vi "Control Panel.vi"(8 "error in (no error)":errorcluster, 11 "Spectrometer Triax 550 in":refnum<class "Spectrometer Triax 550.lvclass">) -> (0 "error out":errorcluster, 3 "Spectrometer Triax 550 out":refnum<class "Spectrometer Triax 550.lvclass">)   [LabVIEW 2023, in "Spectrometer Triax 550.lvclass"]
uses:
  Spectrometer Triax 550.lvclass
  JY-SPEX-TRIAX/controls.llb/Turret Position (TRIAX).ctl
  <vilib>/Utility/error.llb/DialogType.ctl
  JY-SPEX-TRIAX/controls.llb/Slits.ctl
  Spectrometer Triax 550.lvclass/Spectrometer Triax 550.ctl
  JY-SPEX-TRIAX/JY-SPEX-TRIAX.lvlib
  Utility Classes/Scannable/Scannable.lvclass
panel:
  out "?":bool
  out "Title 2":string="Spectrometer Control Program"
  in  "Select Grating":T1
  out "Construct":bool
  out "Init":T2
  out "Status":string
  in  "Shutter":bool
  in  "Set Mirror":bool
  in  "Exit Mirror Pos":bool=TRUE
  in  "Exit":bool
  out "Ready (when flashing)":bool
  out "Slits Open?":bool
  in  "Close Slits":bool
  in  "stepsize":dbl[unit]
  in  "Optimize":bool
  out "groovedensity":dbl[unit] caption="Groove Density"
  out "blazewave":dbl[unit] caption="Blaze Wavelength"
  in  "Set Turret":bool
  out "Title":string="Spectrometer Control Program"
  in  "Reset":bool
  out "Current Wavelength":dbl[unit]
  in  "Target Wavelength":dbl[unit]=4.0000000000000003e-07 min=0.0 max=1.4000000000000001e-06 step=1.0000000000000002e-10
  in  "Jump To Wavelength":bool
  in  "Set Slits":bool
  out "currentlat":dbl[unit] format="%#_6f"
  out "currentaxial":dbl[unit] format="%#_6f"
  in  "gotolat":dbl[unit] min=0.0 max=0.0022 step=1e-05
  in  "gotoaxial":dbl[unit] min=0.0 max=0.0022 step=1e-05 format="%#_6f"
  # "Grating A"
  # "Initialization"
  # "Wavelength Control"
  # "Turret and Other Specs\n(initial mirror value may be incorrect!)"
  # "Grating B"
  # "Slit Widths"
  # "Target"
  # "Current"
  # "AXIAL/CCD"
  # "LATERAL/PMT"
  # "Axial Entrance"
  # "Lateral Exit"
  # "(will round to nearest step size - 2 µm)"
  # "Grating C"
  # "NOTE: initial shutter value may be incorrect!  Toggle switch to set a definite value."
  # "Grooves/mm       Blaze           Cal Offset\nGrating A           1200           500 nm            -35571\nGrating B           1200           750 nm            -38317\nGrating C             600         1000 nm           -40000 (??)"
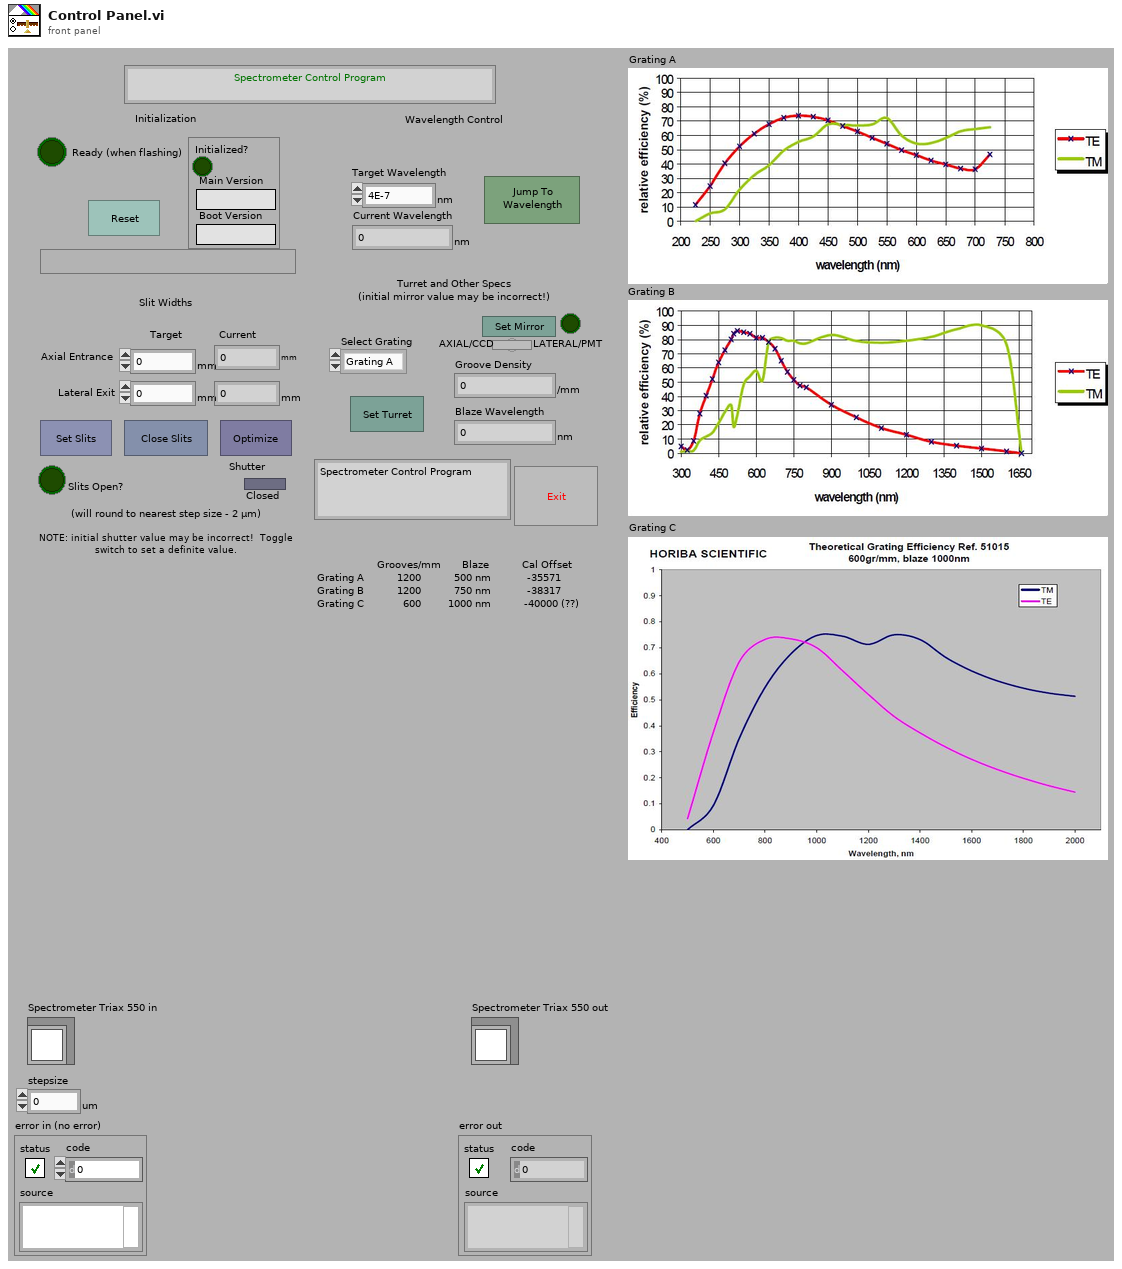
[diagram p1: front panel]
types:
  T1 = typedef "JY-SPEX-TRIAX.lvlib/Turret Position (TRIAX).ctl" = enum16{"Grating A", "Grating B", "Grating C"}
  T2 = cluster{"Initialized?":bool, "Main Version":string, "Boot Version":string, "Spectrometer Number":enum16{"Zero", "One"}}
  T3 = typedef "JY-SPEX-TRIAX.lvlib/Slits.ctl" = enum16{"0 (Front/Axial Entrance)", "1 (Side/Lateral Entrance)", "2 (Front/Axial Exit)", "3 (Side/Lateral Exit)"}
  T4 = typedef "DialogType.ctl" = u16
  T5 = typedef "JY-SPEX-TRIAX.lvlib/Monochromator System Number.ctl" = enum16{"Zero", "One"}
  T6 = cluster{"Initialized?":bool, "Main Version":string, "Boot Version":string, "Mono System #":T5}
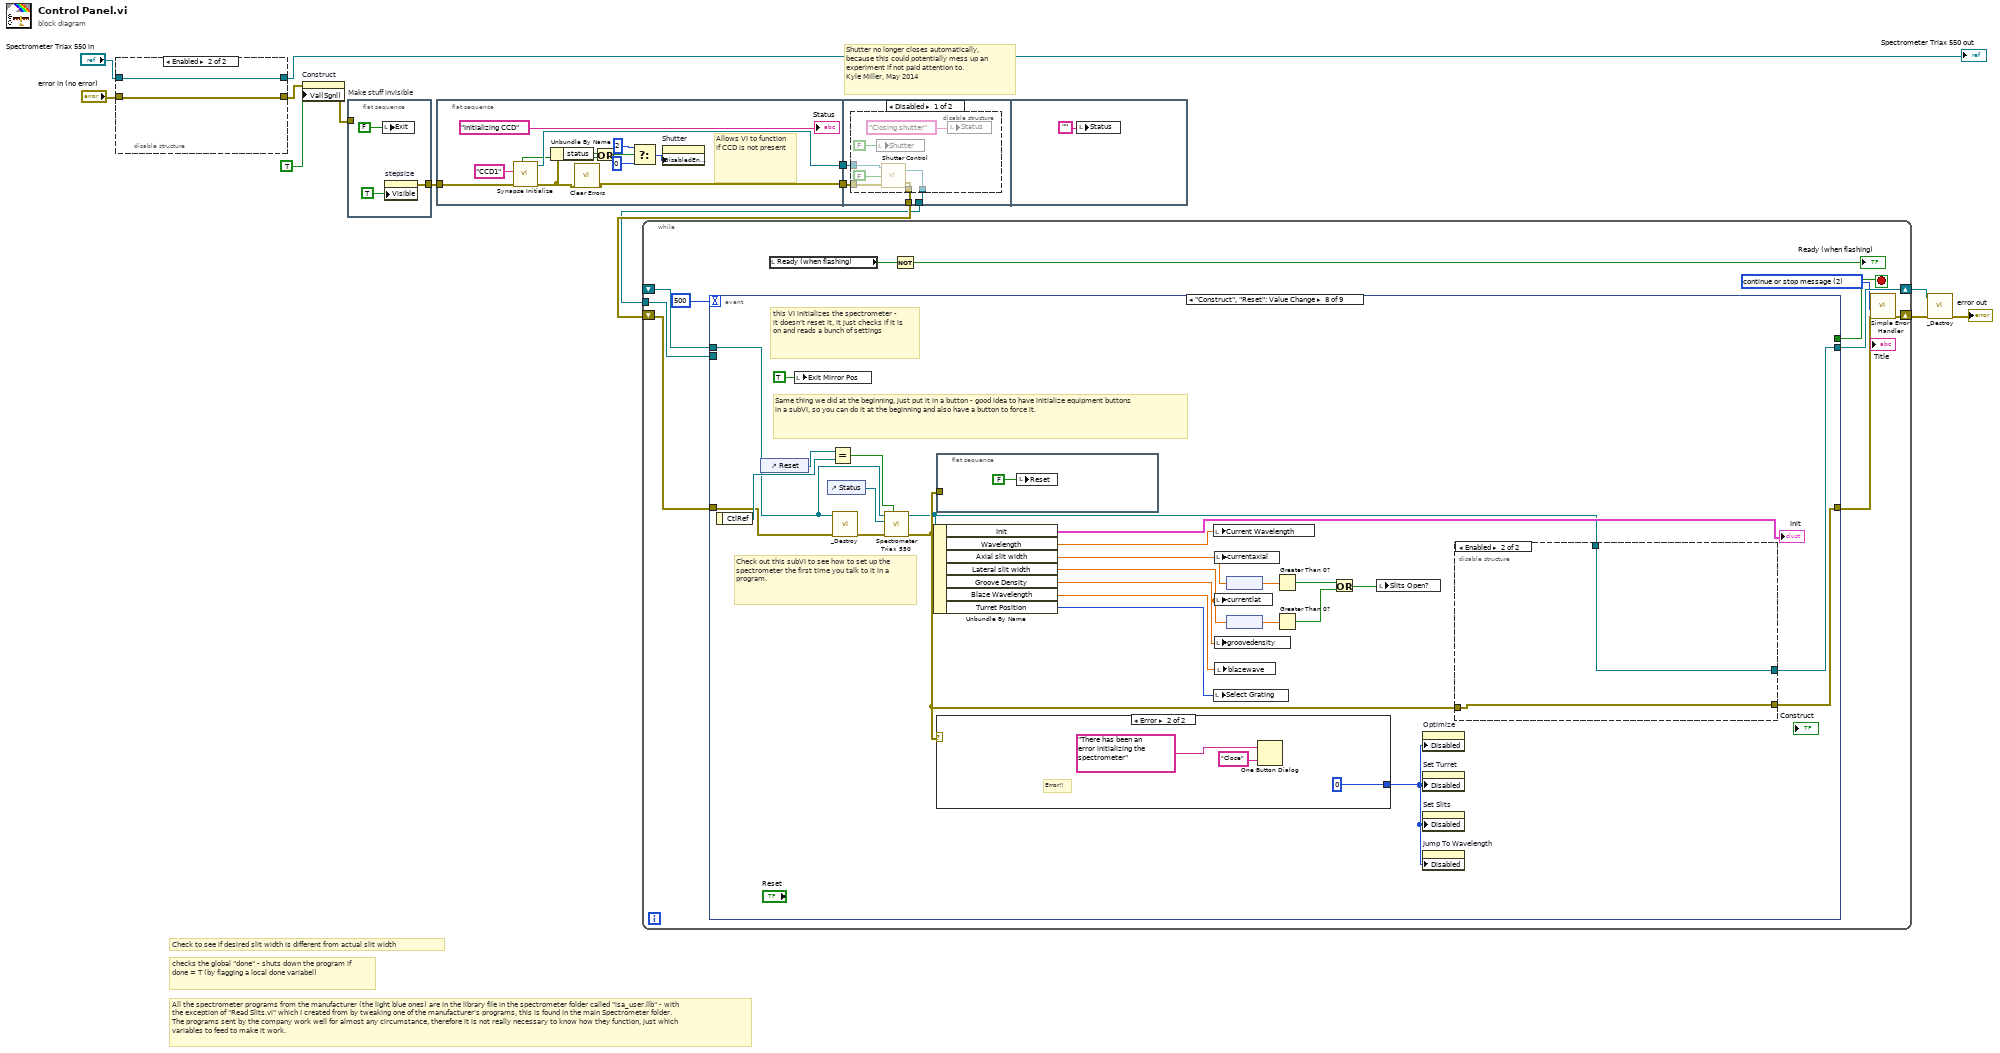
[diagram p0: block diagram]
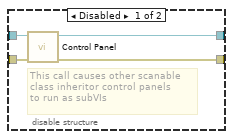
[diagram p2: hidden frame]
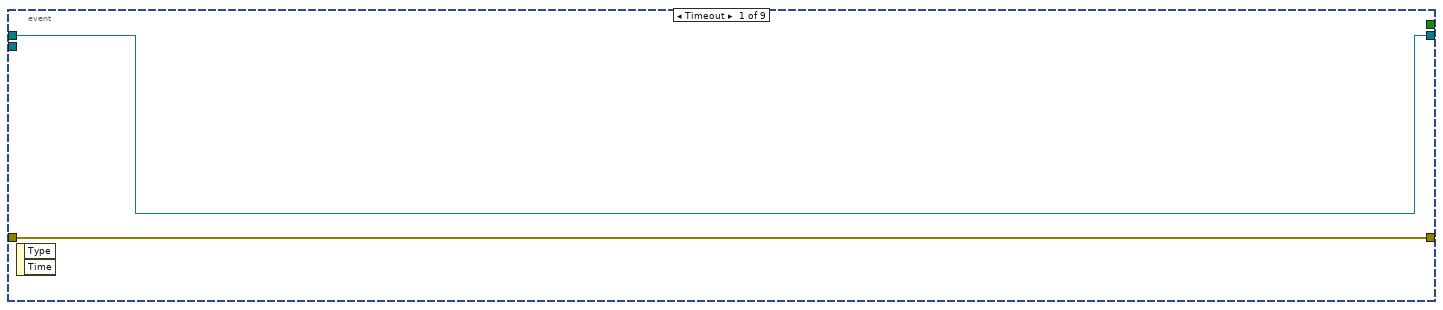
[diagram p4: hidden frame]
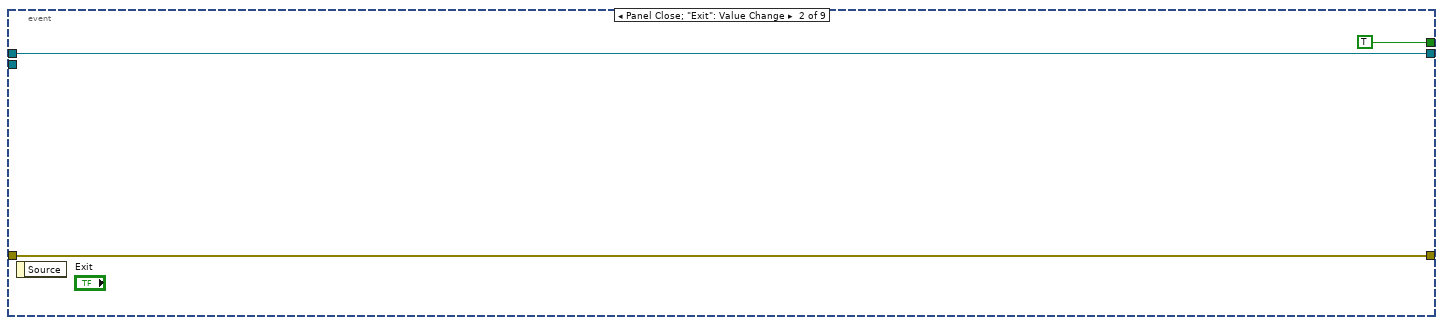
[diagram p5: hidden frame]
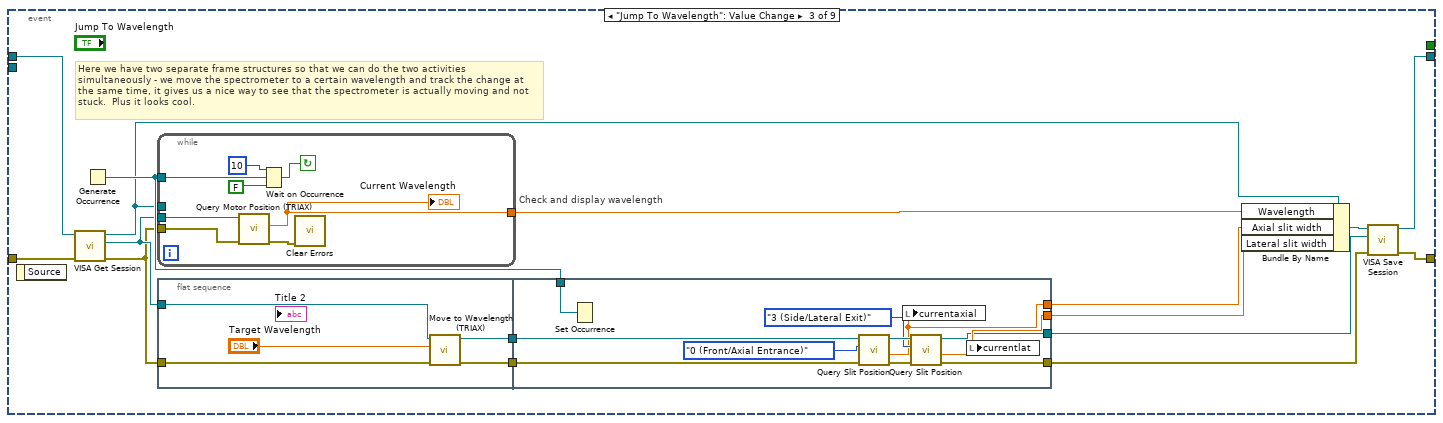
[diagram p6: hidden frame]
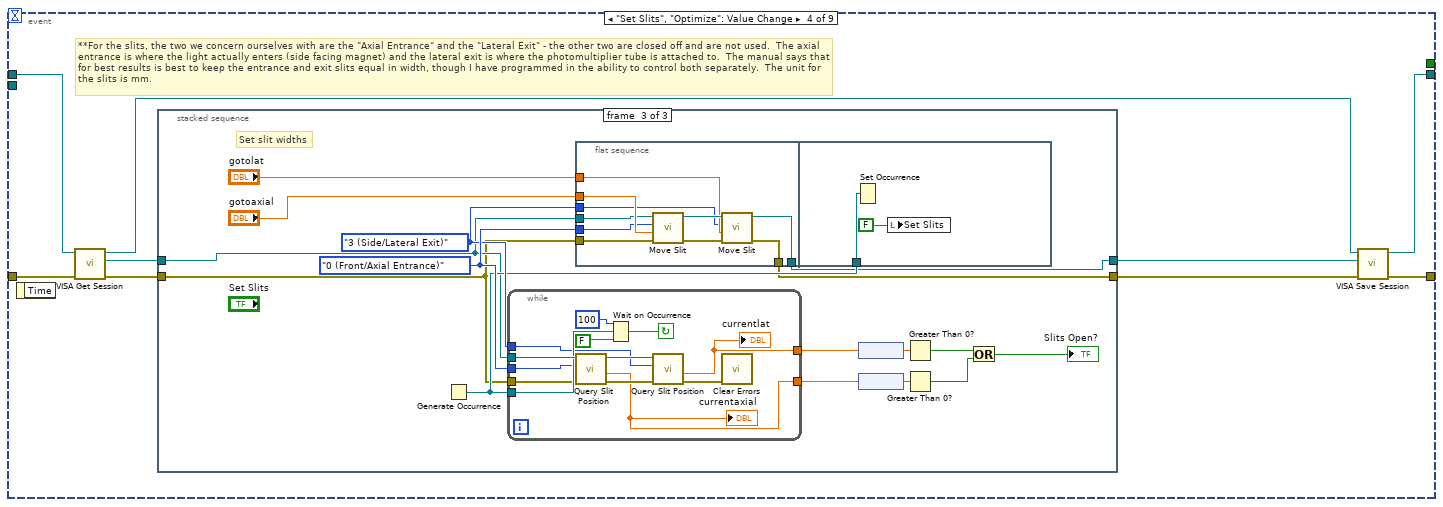
[diagram p7: hidden frame]
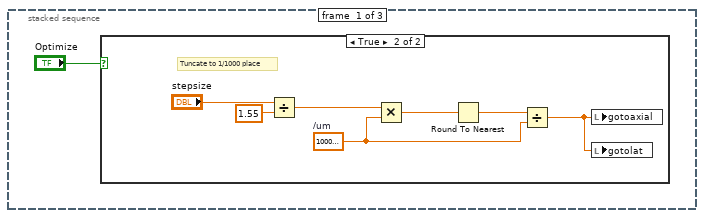
[diagram p8: hidden frame]
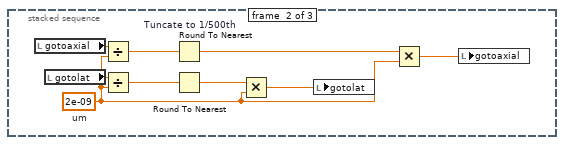
[diagram p10: hidden frame]
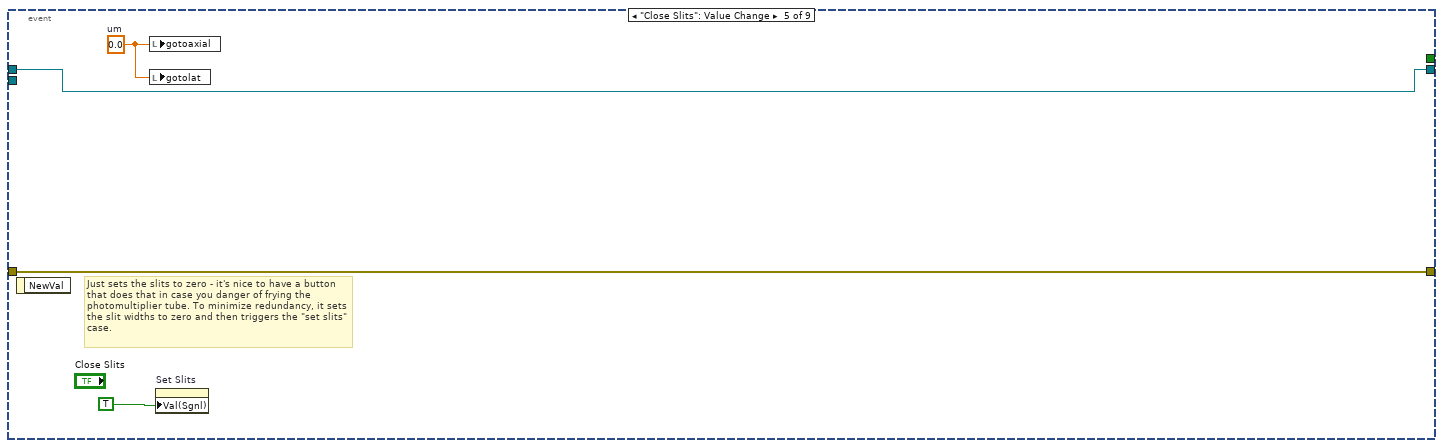
[diagram p11: hidden frame]
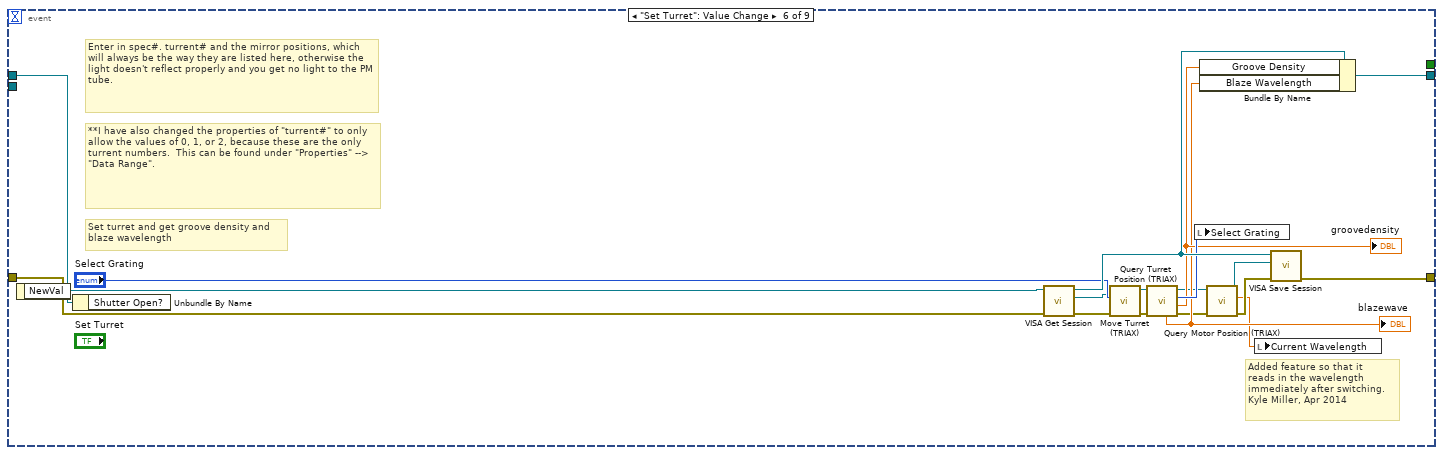
[diagram p12: hidden frame]
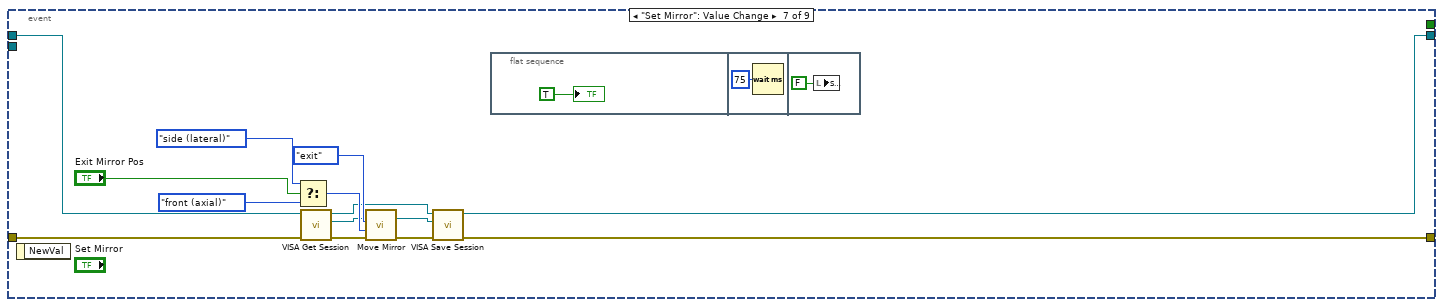
[diagram p13: hidden frame]
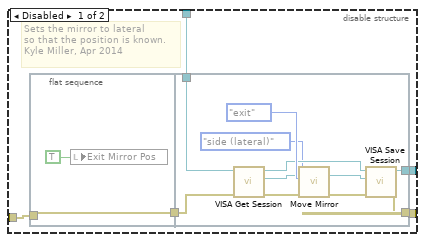
[diagram p14: hidden frame]
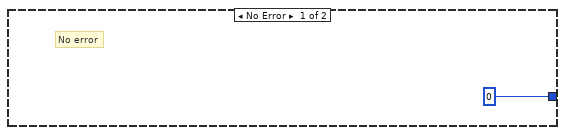
[diagram p15: hidden frame]
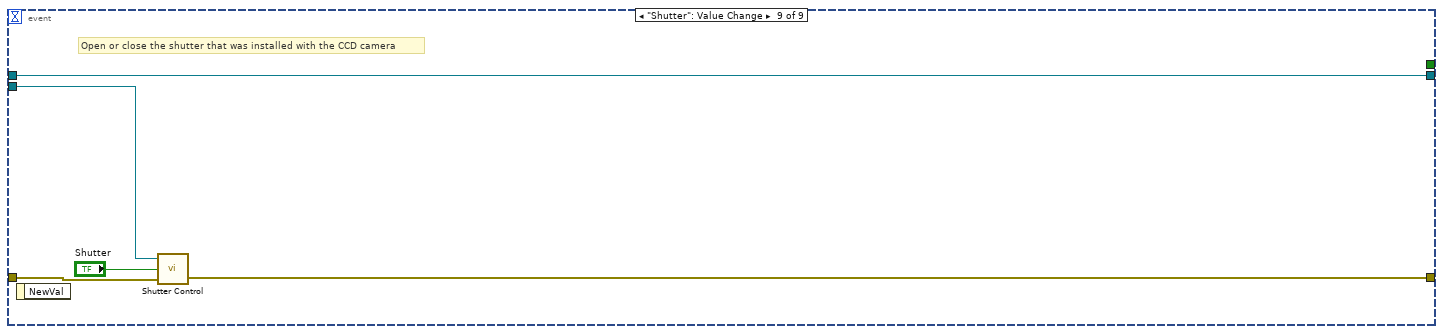
[diagram p16: hidden frame]
diagram:
  # "Shutter no longer closes automatically, because this could potentially mess up an experiment if not paid attention to.\nKyle Miller, May 2014"
  # "Check to see if desired slit width is different from actual slit width"
  # "checks the global \"done\" - shuts down the program if done = T (by flagging a local done variabel)"
  # "All the spectrometer programs from the manufacturer (the light blue ones) are in the library file in the spectrometer folder called \"isa_user.llb\" - with the exception of \"Read Slits.vi\" which I created from by tweaking one of the manufacturer's programs, this is found in the main Spectrometer folder.  The programs sent by the company work well for almost any circumstance, therefore it is not really necessary to know how they function, just which variables to feed to make it work."
  n1 = disable-structure shown="Enabled" {
    disable-tunnel: "error in (no error)" -> [w18 w19]
    disable-tunnel: [w17 w19] -> w13
    disable-tunnel: "Spectrometer Triax 550 in" -> [w16 w20]
    disable-tunnel: [w15 w20] -> w11
    frame Disabled {
      # "This call causes other scanable\nclass inheritor control panels\nto run as subVIs"
      n2 = call-parent "Control Panel.vi"("error in (no error)"=w18, "Instrument in"=w16) -> ("error out"=w17:errorcluster, "Instrument out"=w15:refnum<class "Spectrometer Triax 550.lvclass">)  [unwired: 8 out]
    }
    frame Enabled {
    }
  }
  "Spectrometer Triax 550 out" <- w11
  n3 = property on="Construct" class="Bool (strict)"(error in=w13, "Val(Sgnl)"=TRUE ("Value (Signaling)")) -> (error out=w8:errorcluster)  [unwired: 1 in, 1 out]
  n4 = flat-sequence "Make stuff invisible" {
    tunnel: w8 -> [_]
    tunnel: [w22] -> w3
    frame #0 {
      n5 = local write "Exit"(FALSE ("exit")) -> ()
      n6 = property on="stepsize" class="DigNum (strict)"("Visible"=TRUE) -> (error out=w22:errorcluster)  [unwired: 2 in, 1 out]
    }
  }
  n7 = flat-sequence {
    tunnel: w3 -> [w34]
    tunnel: [w27] -> w2
    tunnel: [w32] -> w1
    tunnel: [w39] -> w5
    tunnel: [w38] -> w4
    tunnel: w2 -> [w37]
    tunnel: w1 -> [w36]
    frame #0 {
      # "Allows VI to function\nif CCD is not present"
      n8 = call "Synapse Initialize.vi"("error in (no error)"=w34, "Unique id"="CCD1") -> ("error out"=w28:errorcluster, "JYCCDLib.IJYCCDReqd"=w32:refnum<k7>, "Disable shutter?"=w25:bool)  [unwired: 1 in, 6 out]
      n9 = Unbundle By Name(w28) -> ("status"=w26:bool)
      n10 = call <vilib>:"Clear Errors.vi"("error in (no error)"=w28) -> ("error out"=w27:errorcluster)  [unwired: 5 in, 1 out]
      n11 = Or(x=w26, y=w25) -> (x .or. y?=w24:bool)
      n12 = Select(t=2, s=w24, f=0) -> (s? t:f=w29:i32)
      n13 = property on="Shutter" class="Bool (strict)"("DisabledEnum"=w29) -> ()  [unwired: 2 in, 2 out]
      "Status" <- "Initializing CCD" ("initialization progress")
    }
    frame #1 {
      n14 = disable-structure shown="Disabled" {
        disable-tunnel: [w44 w47] -> w39
        disable-tunnel: [w43 w48] -> w38
        disable-tunnel: w37 -> [w42 w47]
        disable-tunnel: w36 -> [w41 w48]
        frame Disabled {
          n15 = local write "Shutter"(FALSE ("shutter")) -> ()
          n16 = call "Shutter Control.vi"("input error"=w42, "Shutter"=FALSE, "JYCCDLib.IJYCCDReqd"=w41) -> ("error out"=w44:errorcluster, "JYCCDLib.IJYCCDReqd 2"=w43:refnum<k7>)
          n17 = local write "Status"("Closing shutter" ("initialization progress")) -> ()
        }
        frame Enabled {
        }
      }
    }
    frame #2 {
      n18 = local write "Status"("") -> ()
    }
  }
  n19 = while {
    tunnel: w4 -> [w52]
    shift-right: [w54] -> w6
    shift-left: _ -> [w56]
    shift-right: [w51] -> w7
    shift-left: w5 -> [w55]
    stop <- w60 stop-if-true
    w50 = T4 2 items=["no dialog", "OK message", "continue or stop message", "OK message + warnings", "continue/stop + warnings"] ("type of dialog (OK msg:1)")
    n20 = event shown="[7] \"Construct\", \"Reset\": Value Change" {
      selector: _ -> [_ _ _ _ _ _ _ _ _]
      dyn-events: _ -> [_ _ _ _ _ _ _ _ _]
      timeout: 500 -> [_ _ _ _ _ _ _ _ _]
      tunnel: [_ TRUE _ _ _ _ _ _ _] -> w60
      tunnel: w52 -> [_ _ _ _ _ _ _ _ w266]
      tunnel: [w61 w64 w76 w112 w175 w194 w196 w212 w264] -> w54
      tunnel: w56 -> [w61 w64 w75 w107 w175 w193 w202 w218 w264]
      tunnel: [w62 w63 w66 w111 w173 w180 w195 w214 w262] -> w53
      tunnel: w55 -> [w62 w63 w67 w114 w173 w186 w203 w216 w263]
      event Timeout {
        n21 = event-data() -> ()  [unwired: 3 out]
      }
      event Panel Close; "Exit": Value Change {
        n22 = event-data() -> ()  [unwired: 2 out]
      }
      event "Jump To Wavelength": Value Change {
        # "Here we have two separate frame structures so that we can do the two activities simultaneously - we move the spectrometer to a certain wavelength and track the change at the same time, it gives us a nice way to see that the spectrometer is actually moving and not stuck.  Plus it looks cool."
        n23 = event-data() -> ()  [unwired: 2 out]
        n24 = call-dynamic "VISA Get Session.vi"("error in (no error)"=w67, "Instrument.lvclass in"=w75) -> ("error out"=w68:errorcluster, "VISA Resource Name"=w69:refnum<visa-resource-name>, "Instrument.lvclass out"=w74:refnum<class "Spectrometer Triax 550.lvclass">)  [unwired: 7 out]
        n25 = Generate Occurrence() -> (w78:refnum<k4>)
        n26 = while "Check and display wavelength" {
          tunnel: w74 -> [_]
          tunnel: [w98] -> w81
          tunnel: w78 -> [w103]
          tunnel: w69 -> [w101]
          tunnel: w68 -> [w99]
          stop <- w105 continue-if-true
          n27 = call "Query Motor Position (TRIAX).vi"("error in (no error)"=w99, "VISA resource name"=w101) -> ("error out"=w100:errorcluster, "wavelength"=w98:dbl[unit])  [unwired: 1 in, 7 out]
          "Current Wavelength" <- w98
          n28 = Wait on Occurrence(1:FALSE ("ignore previous (T)"), 2:w103, 3:10 ("ms timeout (-1)")) -> (0:w105:bool)
          n29 = call <vilib>:"Clear Errors.vi"("error in (no error)"=w100) -> ()  [unwired: 1 in, 6 out]
        }
        n30 = flat-sequence {
          tunnel: w69 -> [w86]
          tunnel: [w85] -> w73
          tunnel: [w84] -> w72
          tunnel: w68 -> [w83]
          tunnel: [w87] -> w80
          tunnel: [w92] -> w79
          tunnel: w78 -> [w97]
          tunnel: w73 -> [w95]
          tunnel: w72 -> [w94]
          tunnel: [w90] -> w71
          tunnel: [w89] -> w70
          frame #0 {
            n31 = call "Move to Wavelength (TRIAX).vi"("error in (no error)"=w83, "Target wavelength"="Target Wavelength", "VISA resource name"=w86) -> ("error out"=w84:errorcluster, "VISA resource name out"=w85:refnum<visa-resource-name>)  [unwired: 1 in, 6 out]
          }
          frame #1 {
            n32 = Set Occurrence(w97) -> ()
            n33 = call "Query Slit Position.vi"("error in (no error)"=w94, "Slit (Front/Axial Entrance)"=Slits."0 (Front/Axial Entrance)", "VISA resource name"=w95) -> ("error out"=w88:errorcluster, "Slit Position"=w87:dbl[unit], "VISA resource name out"=w96:refnum<visa-resource-name>)  [unwired: 1 in, 5 out]
            n34 = local write "currentaxial"(w87) -> ()
            n35 = call "Query Slit Position.vi"("error in (no error)"=w88, "Slit (Front/Axial Entrance)"=Slits."3 (Side/Lateral Exit)", "VISA resource name"=w96) -> ("error out"=w89:errorcluster, "Slit Position"=w92:dbl[unit], "VISA resource name out"=w90:refnum<visa-resource-name>)  [unwired: 1 in, 5 out]
            n36 = local write "currentlat"(w92) -> ()
          }
        }
        n37 = Bundle By Name(cluster=w74, "Wavelength"=w81, "Axial slit width"=w80, "Lateral slit width"=w79) -> (w77:refnum<class "Spectrometer Triax 550.lvclass">)
        n38 = call-dynamic "VISA Save Session.vi"("error in (no error)"=w70, "VISA Resource Name"=w71, "Instrument.lvclass in"=w77) -> ("error out"=w66:errorcluster, "Instrument.lvclass out"=w76:refnum<class "Spectrometer Triax 550.lvclass">)  [unwired: 7 out]
      }
      event "Set Slits", "Optimize": Value Change {
        # "**For the slits, the two we concern ourselves with are the \"Axial Entrance\" and the \"Lateral Exit\" - the other two are closed off and are not used.  The axial entrance is where the light actually enters (side facing magnet) and the lateral exit is where the photomultiplier tube is attached to.  The manual says that for best results is best to keep the entrance and exit slits equal in width, though I have programmed in the ability to control both separately.  The unit for the slits is mm."
        n39 = event-data() -> ()  [unwired: 2 out]
        n40 = call-dynamic "VISA Get Session.vi"("error in (no error)"=w114, "Instrument.lvclass in"=w107) -> ("error out"=w113:errorcluster, "VISA Resource Name"=w108:refnum<visa-resource-name>, "Instrument.lvclass out"=w106:refnum<class "Spectrometer Triax 550.lvclass">)  [unwired: 7 out]
        n41 = stacked-sequence {
          tunnel: [_ _ w135] -> w110
          tunnel: w113 -> [_ _ w132]
          tunnel: [_ _ w134] -> w109
          tunnel: w108 -> [_ _ w133]
          frame #0 {
            n42 = case shown="True" "Optimize" {
              frame False {
              }
              frame True {
                w120 = dbl[unit] 1000000000.0  # /um
                # "Tuncate to 1/1000 place"
                n43 = Divide(x="stepsize", y=1.55) -> (x/y=w122:dbl[unit])
                n44 = Multiply(x=w122, y=w120) -> (x*y=w121:dbl)
                n45 = Round To Nearest(number=w121) -> (nearest integer value=w119:dbl)
                n46 = Divide(x=w119, y=w120) -> (x/y=w116:dbl[unit])
                n47 = local write "gotoaxial"(w116) -> ()
                n48 = local write "gotolat"(w116) -> ()
              }
            }
          }
          frame #1 {
            w127 = dbl[unit] 2e-09  # um
            n49 = local read "gotoaxial"() -> (w129:dbl[unit])
            n50 = local read "gotolat"() -> (w128:dbl[unit])
            n51 = Divide(x=w129, y=w127) -> (x/y=w126:dbl)
            n52 = Divide(x=w128, y=w127) -> (x/y=w124:dbl)
            n53 = Round To Nearest "Tuncate to 1/500th"(number=w126) -> (nearest integer value=w125:dbl)
            n54 = Round To Nearest(number=w124) -> (nearest integer value=w123:dbl)
            n55 = Multiply(x=w123, y=w127) -> (x*y=w130:dbl[unit])
            n56 = local write "gotolat"(w130) -> ()
            n57 = Multiply(x=w125, y=w127) -> (x*y=w131:dbl[unit])
            n58 = local write "gotoaxial"(w131) -> ()
          }
          frame #2 {
            w137 = Slits."3 (Side/Lateral Exit)" ("Slit (Front/Axial Entrance)")
            w138 = Slits."0 (Front/Axial Entrance)" ("Slit (Front/Axial Entrance)")
            # "Set slit widths"
            n59 = Generate Occurrence() -> (w136:refnum<k4>)
            n60 = while {
              tunnel: w133 -> [w171]
              tunnel: [w168] -> w140
              tunnel: [w167] -> w139
              tunnel: w136 -> [w166]
              tunnel: w132 -> [w163]
              tunnel: w138 -> [w162]
              tunnel: w137 -> [w161]
              stop <- w164 continue-if-true
              n61 = call "Query Slit Position.vi"("error in (no error)"=w163, "Slit (Front/Axial Entrance)"=w162, "VISA resource name"=w171) -> ("error out"=w170:errorcluster, "Slit Position"=w168:dbl[unit], "VISA resource name out"=w172:refnum<visa-resource-name>)  [unwired: 1 in, 5 out]
              "currentaxial" <- w168
              n62 = Wait on Occurrence(1:FALSE ("ignore previous (T)"), 2:w166, 3:100 ("ms timeout (-1)")) -> (0:w164:bool)
              n63 = call "Query Slit Position.vi"("error in (no error)"=w170, "Slit (Front/Axial Entrance)"=w161, "VISA resource name"=w172) -> ("error out"=w169:errorcluster, "Slit Position"=w167:dbl[unit])  [unwired: 1 in, 6 out]
              "currentlat" <- w167
              n64 = call <vilib>:"Clear Errors.vi"("error in (no error)"=w169) -> ()  [unwired: 1 in, 6 out]
            }
            n65 = flat-sequence {
              tunnel: "gotoaxial" -> [w156]
              tunnel: "gotolat" -> [w155]
              tunnel: w133 -> [w153]
              tunnel: w132 -> [w152]
              tunnel: w138 -> [w151]
              tunnel: w137 -> [w150]
              tunnel: [w148] -> w135
              tunnel: [w149] -> w134
              tunnel: w136 -> [w159]
              frame #0 {
                n66 = call "Move Slit.vi"("error in (no error)"=w152, "Desired Slit Position"=w156, "Slit (Front/Axial Entrance)"=w151, "VISA resource name"=w153) -> ("error out"=w154:errorcluster, "VISA resource name out"=w157:refnum<visa-resource-name>)  [unwired: 1 in, 5 out]
                n67 = call "Move Slit.vi"("error in (no error)"=w154, "Desired Slit Position"=w155, "Slit (Front/Axial Entrance)"=w150, "VISA resource name"=w157) -> ("error out"=w148:errorcluster, "VISA resource name out"=w149:refnum<visa-resource-name>)  [unwired: 1 in, 5 out]
              }
              frame #1 {
                n68 = Set Occurrence(w159) -> ()
                n69 = local write "Set Slits"(FALSE ("Move Slits")) -> ()
              }
            }
            n70 = node(w139) -> (w147:dbl)
            n71 = node(w140) -> (w146:dbl)
            n72 = Greater Than 0?(x=w147) -> (x > 0?=w143:bool)
            n73 = Greater Than 0?(x=w146) -> (x > 0?=w144:bool)
            n74 = Or(x=w143, y=w144) -> (x .or. y?=→"Slits Open?":bool)
          }
        }
        n75 = call-dynamic "VISA Save Session.vi"("error in (no error)"=w110, "VISA Resource Name"=w109, "Instrument.lvclass in"=w106) -> ("error out"=w111:errorcluster, "Instrument.lvclass out"=w112:refnum<class "Spectrometer Triax 550.lvclass">)  [unwired: 7 out]
      }
      event "Close Slits": Value Change {
        w176 = dbl[unit] 0.0  # um
        # "Just sets the slits to zero - it's nice to have a button that does that in case you danger of frying the photomultiplier tube. To minimize redundancy, it sets the slit widths to zero and then triggers the \"set slits\" case."
        n76 = event-data() -> ()  [unwired: 2 out]
        n77 = local write "gotoaxial"(w176) -> ()
        n78 = local write "gotolat"(w176) -> ()
        n79 = property on="Set Slits" class="Bool (strict)"("Val(Sgnl)"=TRUE ("Value (Signaling)")) -> ()  [unwired: 2 in, 2 out]
      }
      event "Set Turret": Value Change {
        # "Added feature so that it\nreads in the wavelength\nimmediately after switching.\nKyle Miller, Apr 2014"
        # "**I have also changed the properties of \"turrent#\" to only allow the values of 0, 1, or 2, because these are the only turrent numbers.  This can be found under \"Properties\" --> \"Data Range\"."
        # "Enter in spec#. turrent# and the mirror positions, which will always be the way they are listed here, otherwise the light doesn't reflect properly and you get no light to the PM tube."
        # "Set turret and get groove density and \nblaze wavelength"
        n80 = event-data() -> ()  [unwired: 2 out]
        n81 = Unbundle By Name(w193) -> ()  [unwired: 1 out]
        n82 = call-dynamic "VISA Get Session.vi"("error in (no error)"=w186, "Instrument.lvclass in"=w193) -> ("error out"=w187:errorcluster, "VISA Resource Name"=w188:refnum<visa-resource-name>, "Instrument.lvclass out"=w192:refnum<class "Spectrometer Triax 550.lvclass">)  [unwired: 7 out]
        n83 = call "Move Turret (TRIAX).vi"("error in (no error)"=w187, "turret position (0)"="Select Grating", "VISA resource name"=w188) -> ("error out"=w189:errorcluster, "VISA resource name out"=w190:refnum<visa-resource-name>)  [unwired: 1 in, 6 out]
        n84 = call "Query Turret Position (TRIAX).vi"("error in (no error)"=w189, "VISA resource name"=w190) -> ("error out"=w182:errorcluster, "Groove Density"=w184:dbl[unit], "Turret Position"=w185:T1, "VISA resource name out"=w179:refnum<visa-resource-name>, "Blaze Wavelength"=w183:dbl[unit])  [unwired: 1 in, 4 out]
        "blazewave" <- w183
        "groovedensity" <- w184
        n85 = local write "Select Grating"(w185) -> ()
        n86 = Bundle By Name(cluster=w192, "Groove Density"=w184, "Blaze Wavelength"=w183) -> (w194:refnum<class "Spectrometer Triax 550.lvclass">)
        n87 = call "Query Motor Position (TRIAX).vi"("error in (no error)"=w182, "VISA resource name"=w179) -> ("error out"=w181:errorcluster, "wavelength"=w177:dbl[unit], "VISA resource name out"=w178:refnum<visa-resource-name>)  [unwired: 1 in, 6 out]
        n88 = local write "Current Wavelength"(w177) -> ()
        n89 = call-dynamic "VISA Save Session.vi"("error in (no error)"=w181, "VISA Resource Name"=w178, "Instrument.lvclass in"=w192) -> ("error out"=w180:errorcluster)  [unwired: 8 out]
      }
      event "Set Mirror": Value Change {
        n90 = event-data() -> ()  [unwired: 2 out]
        n91 = Select(t=enum16{"side (lateral)", "front (axial)"}."side (lateral)" ("position (side/lateral)"), s="Exit Mirror Pos", f=enum16{"side (lateral)", "front (axial)"}."front (axial)" ("position (side/lateral)")) -> (s? t:f=w204:enum16{"side (lateral)", "front (axial)"})
        n92 = call-dynamic "VISA Get Session.vi"("error in (no error)"=w203, "Instrument.lvclass in"=w202) -> ("error out"=w200:errorcluster, "VISA Resource Name"=w201:refnum<visa-resource-name>, "Instrument.lvclass out"=w199:refnum<class "Spectrometer Triax 550.lvclass">)  [unwired: 7 out]
        n93 = call "Move Mirror.vi"("error in (no error)"=w200, "position (side/lateral)"=w204, "mirror (exit)"=enum16{"entrance", "exit"}."exit", "VISA resource name"=w201) -> ("error out"=w198:errorcluster, "VISA resource name out"=w197:refnum<visa-resource-name>)  [unwired: 1 in, 5 out]
        n94 = call-dynamic "VISA Save Session.vi"("error in (no error)"=w198, "VISA Resource Name"=w197, "Instrument.lvclass in"=w199) -> ("error out"=w195:errorcluster, "Instrument.lvclass out"=w196:refnum<class "Spectrometer Triax 550.lvclass">)  [unwired: 7 out]
        n95 = flat-sequence {
          frame #0 {
            "?" <- TRUE ("Mirror set")
          }
          frame #1 {
            n96 = Wait (ms)(milliseconds to wait=u32 75) -> ()  [unwired: 1 out]
          }
          frame #2 {
            n97 = local write item#31(FALSE ("Mirror set")) -> ()
          }
        }
      }
      event "Construct", "Reset": Value Change {
        # "Check out this subVI to see how to set up the spectrometer the first time you talk to it in a program."
        # "this VI initializes the spectrometer - it doesn't reset it, it just checks if it is on and reads a bunch of settings"
        # "Same thing we did at the beginning, just put it in a button - good idea to have initialize equipment buttons in a subVI, so you can do it at the beginning and also have a button to force it."
        n98 = event-data() -> ("CtlRef"=w221:refnum<vi>)  [unwired: 1 out]
        n99 = control-ref of="Reset"() -> (w220:refnum<vi>)
        n100 = local write "Exit Mirror Pos"(TRUE ("Exit Mirror Pos")) -> ()
        n101 = control-ref of="Status"() -> (w223:refnum<vi>)
        n102 = Equal?(x=w220, y=w221) -> (x = y?=w219:bool)
        n103 = call-dynamic "_Destroy.vi"("error in (no error)"=w216, "Instrument in"=w218) -> ("error out"=w217:errorcluster)  [unwired: 9 out]
        n104 = call "Spectrometer Triax 550.vi"("Force Reset? (F)"=w219, "error in (no error)"=w217, "Ref to a Status Box"=w223, "Spectrometer Triax 550 in"=w218) -> ("error out"=w215:errorcluster, "Spectrometer Triax 550 out"=w213:refnum<class "Spectrometer Triax 550.lvclass">)  [unwired: 6 out]
        n105 = Unbundle By Name(w213) -> ("Init"=→"Init":T6, "Wavelength"=w232:dbl[unit], "Axial slit width"=w225:dbl[unit], "Lateral slit width"=w229:dbl[unit], "Groove Density"=w231:dbl[unit], "Blaze Wavelength"=w230:dbl[unit], "Turret Position"=w224:T1)
        n106 = flat-sequence {
          tunnel: w215 -> [_]
          frame #0 {
            n107 = local write "Reset"(FALSE ("initialize")) -> ()
          }
        }
        n108 = case shown="Error" w215 {
          tunnel: [0 0] -> w236
          frame No Error {
            # "No error"
          }
          frame Error {
            # "Error!!"
            n109 = One Button Dialog(message="There has been an error initializing the spectrometer", button name ("OK")="Close") -> ()  [unwired: 1 out]
          }
        }
        n110 = local write "Current Wavelength"(w232) -> ()
        n111 = local write "Select Grating"(w224) -> ()
        n112 = local write "currentaxial"(w225) -> ()
        n113 = local write "currentlat"(w229) -> ()
        n114 = local write "groovedensity"(w231) -> ()
        n115 = local write "blazewave"(w230) -> ()
        n116 = node(w225) -> (w227:dbl)
        n117 = node(w229) -> (w226:dbl)
        n118 = Greater Than 0?(x=w227) -> (x > 0?=w235:bool)
        n119 = Greater Than 0?(x=w226) -> (x > 0?=w234:bool)
        n120 = Or(x=w235, y=w234) -> (x .or. y?=w233:bool)
        n121 = local write "Slits Open?"(w233) -> ()
        n122 = property on="Optimize" class="Bool"("Disabled"=w236) -> ()  [unwired: 2 in, 2 out]
        n123 = property on="Set Turret" class="Bool"("Disabled"=w236) -> ()  [unwired: 2 in, 2 out]
        n124 = property on="Set Slits" class="Bool (strict)"("Disabled"=w236) -> ()  [unwired: 2 in, 2 out]
        n125 = property on="Jump To Wavelength" class="Bool"("Disabled"=w236) -> ()  [unwired: 2 in, 2 out]
        n126 = disable-structure shown="Enabled" {
          disable-tunnel: w215 -> [w240 w255]
          disable-tunnel: [w239 w255] -> w214
          disable-tunnel: w213 -> [w238 w256]
          disable-tunnel: [w237 w256] -> w212
          frame Disabled {
            # "Sets the mirror to lateral\nso that the position is known.\nKyle Miller, Apr 2014"
            n127 = flat-sequence {
              tunnel: w240 -> [w242]
              tunnel: [w242] -> w241
              tunnel: w241 -> [w245]
              tunnel: [w244] -> w239
              tunnel: w238 -> [w248]
              tunnel: [w247] -> w237
              frame #0 {
                n128 = local write "Exit Mirror Pos"(TRUE ("Exit Mirror Pos")) -> ()
              }
              frame #1 {
                n129 = call-dynamic "VISA Get Session.vi"("error in (no error)"=w245, "Instrument.lvclass in"=w248) -> ("error out"=w252:errorcluster, "VISA Resource Name"=w253:refnum<visa-resource-name>, "Instrument.lvclass out"=w251:refnum<class "Spectrometer Triax 550.lvclass">)  [unwired: 7 out]
                n130 = call "Move Mirror.vi"("error in (no error)"=w252, "position (side/lateral)"=enum16{"side (lateral)", "front (axial)"}."side (lateral)", "mirror (exit)"=enum16{"entrance", "exit"}."exit", "VISA resource name"=w253) -> ("error out"=w250:errorcluster, "VISA resource name out"=w249:refnum<visa-resource-name>)  [unwired: 1 in, 5 out]
                n131 = call-dynamic "VISA Save Session.vi"("error in (no error)"=w250, "VISA Resource Name"=w249, "Instrument.lvclass in"=w251) -> ("error out"=w244:errorcluster, "Instrument.lvclass out"=w247:refnum<class "Spectrometer Triax 550.lvclass">)  [unwired: 7 out]
              }
            }
          }
          frame Enabled {
          }
        }
      }
      event "Shutter": Value Change {
        # "Open or close the shutter that was installed with the CCD camera"
        n132 = event-data() -> ()  [unwired: 2 out]
        n133 = call "Shutter Control.vi"("input error"=w263, "Shutter"="Shutter", "JYCCDLib.IJYCCDReqd"=w266) -> ("error out"=w262:errorcluster)  [unwired: 1 out]
      }
    }
    n134 = local read "Ready (when flashing)"() -> (w58:bool)
    n135 = Not(x=w58) -> (.not. x?=→"Ready (when flashing)":bool)
    n136 = call <vilib>:"Simple Error Handler.vi"("type of dialog (OK msg:1)"=w50, "error in (no error)"=w53) -> ("error out"=w51:errorcluster)  [unwired: 7 out]
  }
  n137 = call-dynamic "_Destroy.vi"("error in (no error)"=w7, "Instrument in"=w6) -> ("error out"=→"error out":errorcluster)  [unwired: 9 out]
